vi "ConnectOsc.vi"(8 "error in (no error)":errorcluster, 9 "Command":string, 10 "ON/OFF":bool, 11 "Control in":refnum<class "Control-Server.lvclass">) -> (0 "error out":errorcluster, 3 "Control out":refnum<class "Control-Server.lvclass">)   [LabVIEW 2020, in "Control-Server.lvclass"]
uses:
  Control-Server.lvclass
  dependecies/ControlsVIs/Clusters-def/Message types.ctl
  Control-Server.lvclass/Control-Server.ctl
  Oscilloscope/Oscilloscope.lvclass
  C:/dev/TRANCON/Classes/GeneralFunctionality/GeneralFunctionality.lvclass
  Message/Message.lvclass
  GeneralFunctionality/GeneralFunctionality.lvclass
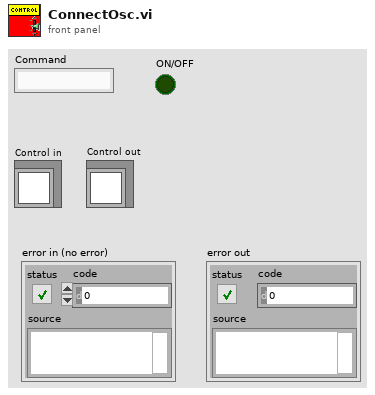
[diagram p1: front panel]
types:
  T1 = typedef "Message types.ctl" = string
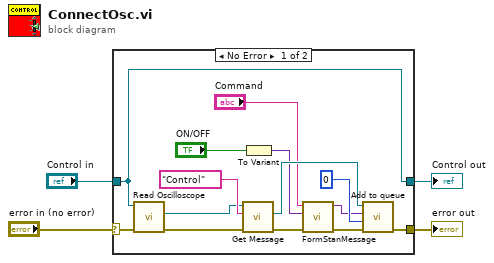
[diagram p0: block diagram]
diagram:
  n1 = case shown="No Error" "error in (no error)" {
    selector: "error in (no error)" -> [w12 w20]
    tunnel: [w13 w19] -> w4
    tunnel: "Control in" -> [w13 w19]
    tunnel: [w14 w20] -> w2
    frame No Error {
      n2 = call "Read Oscilloscope.vi"("error in (no error)"=w12, "Control-Server en entrée"=w13) -> ("error out"=w11:errorcluster, "Oscilloscope.lvclass"=w10:refnum<class "Oscilloscope.lvclass">)  [unwired: 7 in, 1 out]
      n3 = call "Get Message.vi"("error in (no error)"=w11, "Message type"=T1 "Control", "GeneralFunctionality en entrée"=w10) -> ("error out"=w9:errorcluster, "Message.lvclass"=w18:refnum<class "Message.lvclass">)  [unwired: 6 in, 1 out]
      n4 = To Variant(anything="ON/OFF") -> (Variant=w6:variant)
      n5 = call "FormStanMessage.vi"("error in"=w9, "data"=w6, "Command"="Command") -> ("error out"=w8:errorcluster, "message"=w7:variant)  [unwired: 7 in]
      n6 = call "Add to queue.vi"("error in (no error)"=w8, "timeout in ms (-1)"=0, "Data"=w7, "Message in"=w18) -> ("error out"=w14:errorcluster)  [unwired: 6 in, 1 out]
    }
    frame Error {
    }
  }
  "error out" <- w2
  "Control out" <- w4
